vi "main.vi"() -> ()   [LabVIEW 2020]
uses:
  <userlib>/_NEVSTOP/TagDB/TagDB.lvlib
  <userlib>/_NEVSTOP/Communicable State Machine(CSM)/addons/Watchdog/CSM Watchdog.lvlib
  <userlib>/_NEVSTOP/Communicable State Machine(CSM)/Communicable State Machine.lvlib
  <userlib>/_NEVSTOP/Communicable State Machine(CSM)/addons/Logger/CSM File Logger.lvlib
panel:
  in  "Stop":bool
  in  "Play":bool
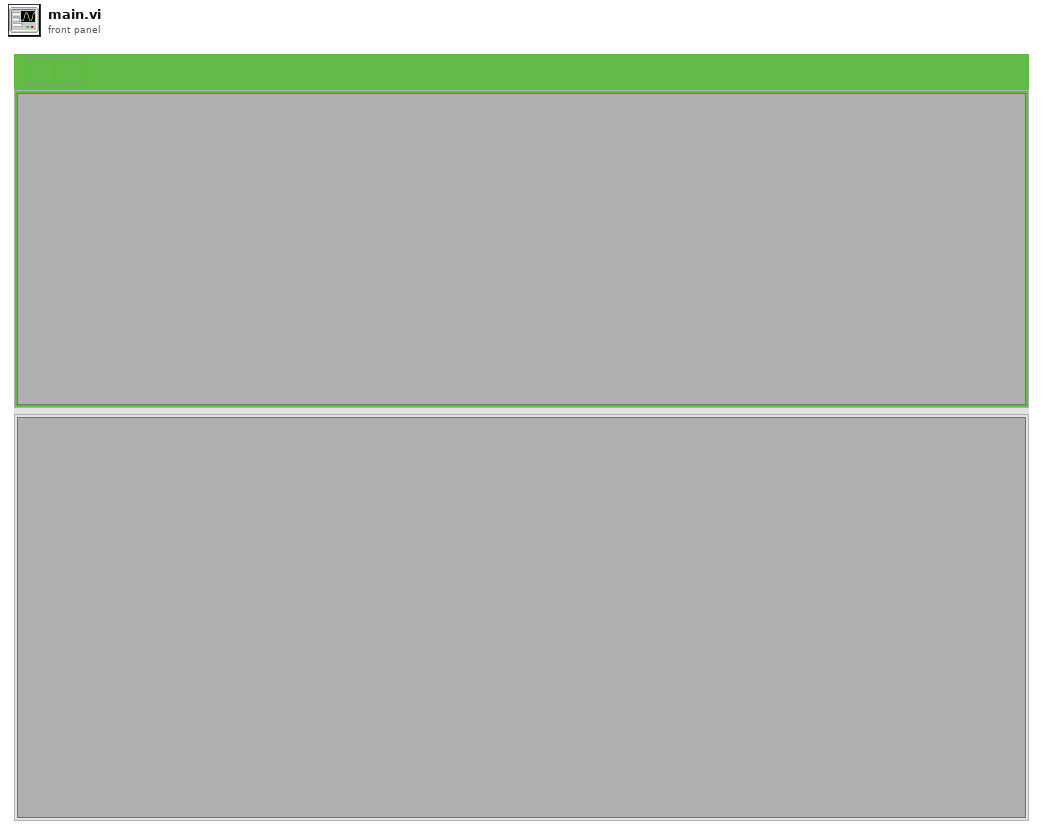
[diagram p1: front panel]
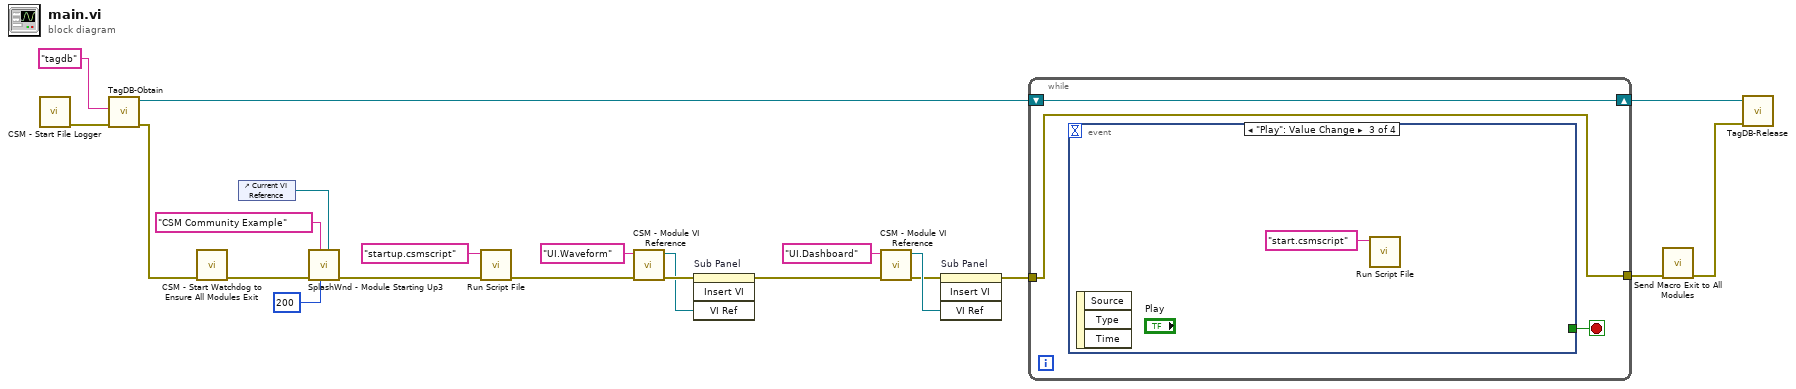
[diagram p0: block diagram]
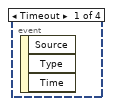
[diagram p2: hidden frame]
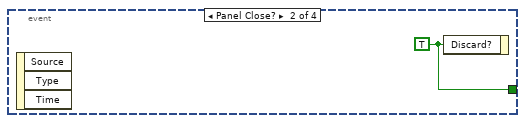
[diagram p3: hidden frame]
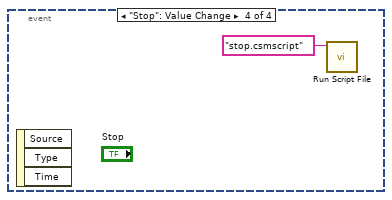
[diagram p4: hidden frame]
diagram:
  n1 = call <userlib>:"CSM - Start File Logger.vi"() -> ("error out"=w2:errorcluster)  [unwired: 9 in, 2 out]
  n2 = call <userlib>:"TagDB-Obtain.vi"("error in (no error)"=w2, "name (unnamed)"="tagdb") -> ("error out"=w18:errorcluster, "TagDB"=w21:refnum<k1>)  [unwired: 3 in, 1 out]
  n3 = call <userlib>:"CSM - Start Watchdog to Ensure All Modules Exit.vi"("error in (no error)"=w18) -> ("error out"=w11:errorcluster)  [unwired: 10 in]
  n4 = control-ref of="Current VI Reference"() -> (w9:refnum<vi>)
  n5 = call "SplashWnd - Module Starting Up3.vi"("Background VI Ref (Callee's Caller)"=w9, "LoadingWait(ms)"=u32 200, "Title"="CSM Community Example", "Error In (No Error)"=w11) -> ("error out"=w10:errorcluster)  [unwired: 7 in]
  n6 = call "Run Script File.vi"("error in (no error)"=w10, "pattern"="startup.csmscript") -> ("error out"=w4:errorcluster)  [unwired: 9 in]
  n7 = call <userlib>:"CSM - Module VI Reference.vi"("error in (no error)"=w4, "CSM Name"="UI.Waveform") -> ("error out"=w6:errorcluster, "CSM Module VIRef"=w5:refnum<vi>)  [unwired: 8 in]
  n8 = invoke on="Sub Panel" class="SubPnl" method="Insert VI"(error in=w6, "VI Ref"=w5) -> (error out=w3:errorcluster)  [unwired: 2 in, 3 out]
  n9 = call <userlib>:"CSM - Module VI Reference.vi"("error in (no error)"=w3, "CSM Name"="UI.Dashboard") -> ("error out"=w16:errorcluster, "CSM Module VIRef"=w17:refnum<vi>)  [unwired: 8 in]
  n10 = invoke on="Sub Panel" class="SubPnl" method="Insert VI"(error in=w16, "VI Ref"=w17) -> (error out=w15:errorcluster)  [unwired: 2 in, 3 out]
  n11 = while {
    shift-right: [w24] -> w20
    shift-left: w21 -> [w24]
    tunnel: w15 -> [w23]
    tunnel: [w23] -> w13
    stop <- w25 stop-if-true
    n12 = event shown="[2] \"Play\": Value Change" {
      selector: _ -> [_ _ _ _]
      dyn-events: _ -> [_ _ _ _]
      timeout: _ -> [_ _ _ _]
      tunnel: [_ w26 _ _] -> w25
      event Timeout {
        n13 = event-data() -> ()  [unwired: 1 in, 3 out]
      }
      event Panel Close? {
        w26 = TRUE ("Discard?")
        n14 = event-data() -> ()  [unwired: 1 in, 3 out]
        n15 = event-data("Discard?"=w26) -> ()  [unwired: 1 in, 1 out]
      }
      event "Play": Value Change {
        n16 = event-data() -> ()  [unwired: 1 in, 3 out]
        n17 = call "Run Script File.vi"("pattern"="start.csmscript") -> ()  [unwired: 10 in, 1 out]
      }
      event "Stop": Value Change {
        n18 = event-data() -> ()  [unwired: 1 in, 3 out]
        n19 = call "Run Script File.vi"("pattern"="stop.csmscript") -> ()  [unwired: 10 in, 1 out]
      }
    }
  }
  n20 = call "Send Macro Exit to All Modules.vi"("error in (no error)"=w13) -> ("error out"=w12:errorcluster)  [unwired: 10 in]
  n21 = call <userlib>:"TagDB-Release.vi"("error in (no error)"=w12, "TagDB"=w20) -> ()  [unwired: 9 in, 1 out]
